vi "RSZVB Set Sweep Time Auto.vi"(8 "error in (no error)":errorcluster {"code" format="%.0x"}, 9 "Auto Sweep Time (T: On)":bool=TRUE, 10 "Channel (1)":i32=1, 11 "VISA session":refnum<visa-resource-name>) -> (0 "error out":errorcluster {"code" format="%.0x"}, 3 "dup VISA session":refnum<visa-resource-name>)   [LabVIEW 2011]
doc: "This VI when enabled, the (minimum) sweep duration is calculated internally using the other channel settings and zero delay ([SENSe<Ch>:]SWEep:DWELl). \n\nNote(s):\n\nThe automatically calculated sweep duration is ignored for the sweep types Time and CW Mode.\n\nRemote-control command(s):\n[SENSe<Ch>:]SWEep:TIME:AUTO <Boolean>"
panel:
  # "On\nOff"
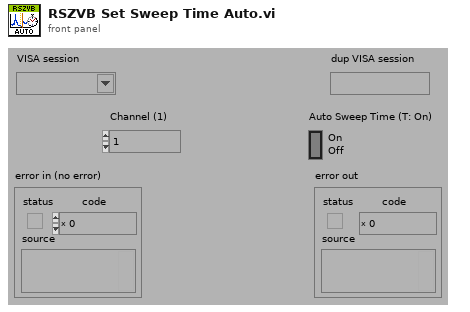
[diagram p1: front panel]
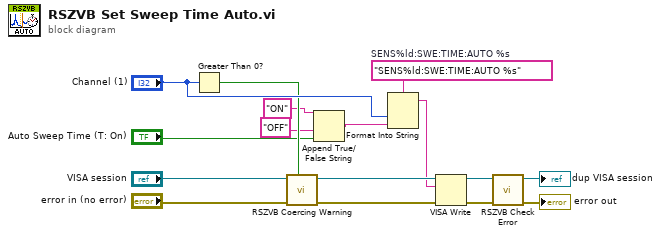
[diagram p0: block diagram]
diagram:
  w16 = "SENS%ld:SWE:TIME:AUTO %s"  # SENS%ld:SWE:TIME:AUTO %s
  n1 = Greater Than 0?(x="Channel (1)") -> (x > 0?=w5:bool)
  n2 = call "RSZVB Coercing Warning.vi"("In Range?"=w5, "error in (no error)"="error in (no error)", "VISA session"="VISA session") -> ("error out"=w14:errorcluster, "dup VISA session"=w15:refnum<visa-resource-name>)  [unwired: 7 in]
  n3 = Append True/False String(1:"Auto Sweep Time (T: On)", 2:"OFF", 3:"ON") -> (0:w2:string)  [unwired: 1 in]
  n4 = Format Into String(format string=w16, "Channel (1)", w2) -> (resulting string=w11:string)  [unwired: 2 in, 1 out]
  n5 = VISA Write(VISA resource name=w15, write buffer=w11, error in (no error)=w14) -> (VISA resource name out=w12:refnum<visa-resource-name>, error out=w13:errorcluster)  [unwired: 1 out]
  n6 = call "RSZVB Check Error.vi"("error in (no error)"=w13, "VISA session"=w12) -> ("error out"=→"error out":errorcluster, "dup VISA session"=→"dup VISA session":refnum<visa-resource-name>)  [unwired: 8 in]
